vi "Read Data.vi"(8 "error in":errorcluster, 11 "M data in":refnum<class "M data.lvclass">) -> (0 "error out":errorcluster, 2 "Data":sgl[](array[numeric]), 3 "M data out":refnum<class "M data.lvclass">)   [LabVIEW 2015, in "M data.lvclass"]
uses:
  M data.lvclass
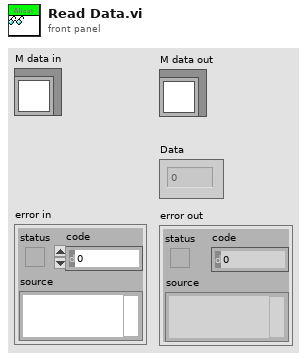
[diagram p1: front panel]
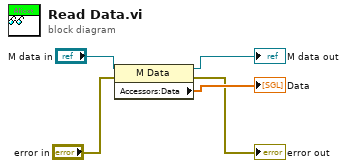
[diagram p0: block diagram]
diagram:
  n1 = property class="M Data"(reference="M data in", error in="error in") -> (reference out=→"M data out":refnum<class "M data.lvclass">, error out=→"error out":errorcluster, "Accessors:Data"=→"Data":sgl[])
